vi "LABVIEW1.vi"() -> ()   [LabVIEW 2019]
panel:
  out "最大値":dbl
  out "波形グラフ":dynamicdata(graph)
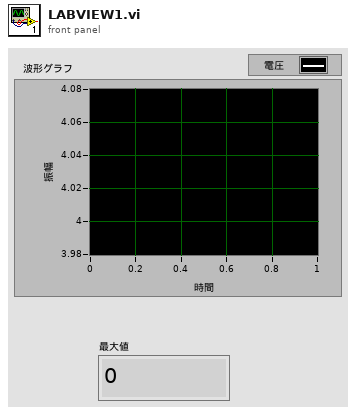
[diagram p1: front panel]
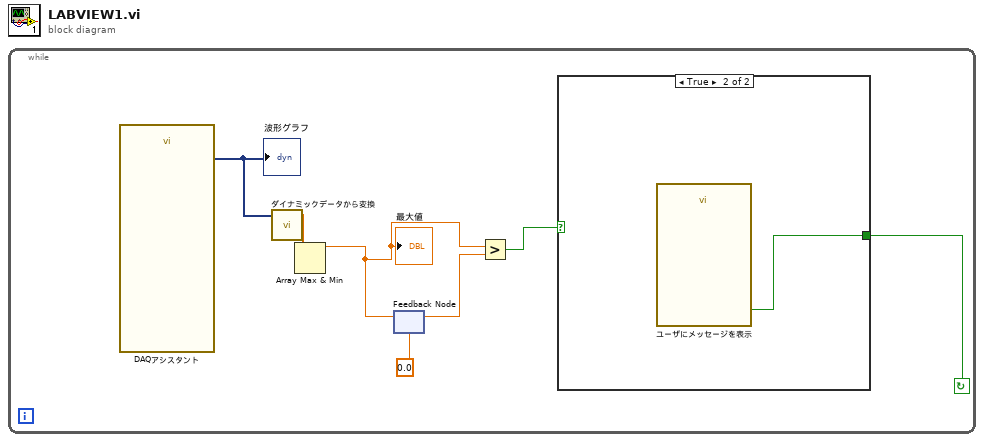
[diagram p0: block diagram]
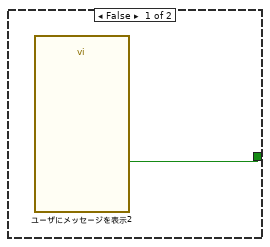
[diagram p2: hidden frame]
diagram:
  n1 = while {
    stop <- w1 continue-if-true
    n2 = call "DAQアシスタント"() -> ("data"=w7:dynamicdata)  [unwired: 17 in, 2 out]
    "波形グラフ" <- w7
    n3 = call "ダイナミックデータから変換"("Dynamic Data Type"=w7) -> ("Array"=w6:dbl[])  [unwired: 3 in]
    n4 = Array Max & Min(array=w6) -> (max value=w5:dbl)  [unwired: 3 out]
    "最大値" <- w5
    n5 = feedback-in #1(w5) -> ()
    n6 = feedback #1(0.0) -> (w4:dbl)
    n7 = Greater?(x=w5, y=w4) -> (0:w2:bool)
    n8 = case shown="TRUE" w2 {
      tunnel: [w8 w9] -> w1
      frame False {
        n9 = call "ユーザにメッセージを表示2"() -> ("続ける"=w8:bool)  [unwired: 10 in, 1 out]
      }
      frame True {
        n10 = call "ユーザにメッセージを表示"() -> ("OK"=w9:bool)  [unwired: 10 in, 1 out]
      }
    }
  }
